vi "FlatSequenceToJSON.vi"(0 "FlatSequence in":refnum<vi>, 1 "Origin Path":path, 5 "Relative Bounds":cluster{"x":i32, "y":i32, "w":i32, "h":i32}, 7 "Current Path":path, 9 "Component Idx":i32, 11 "error in":errorcluster) -> (8 "JSON":string, 15 "error out":errorcluster)   [LabVIEW 2017]
doc: "Converts a flat sequence structure into a JSON"
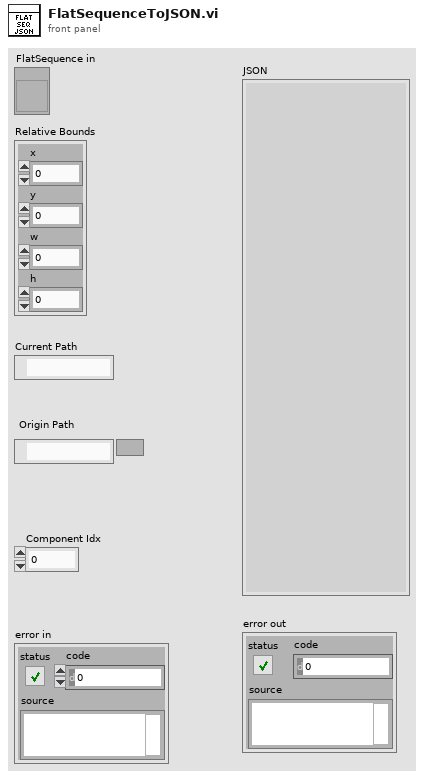
[diagram p1: front panel]
types:
  T1 = typedef "LVRectTypeDef.ctl" = cluster{"Left":i16, "Top":i16, "Right":i16, "Bottom":i16}
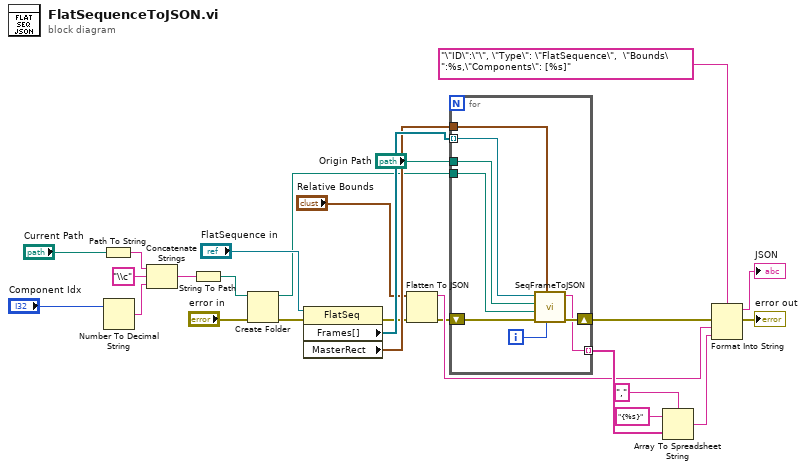
[diagram p0: block diagram]
diagram:
  n1 = Path To String(path="Current Path") -> (string=w15:string)
  n2 = Number To Decimal String(number="Component Idx") -> (decimal integer string=w16:string)  [unwired: 1 in]
  n3 = Concatenate Strings(w15, "\\c" ("string"), w16) -> (w14:string)
  n4 = String To Path(string=w14) -> (path=w13:path)
  n5 = Create Folder(path (use dialog)=w13, error in="error in") -> (created path=w10:path, error out=w11:errorcluster)  [unwired: 1 in, 1 out]
  n6 = property class="FlatSeq"(reference="FlatSequence in", error in=w11) -> (error out=w2:errorcluster, "Frames[]"=w25:refnum<vi>[], "MasterRect"=w20:T1)  [unwired: 1 out]
  n7 = Flatten To JSON(anything="Relative Bounds", error in (no error)=w2) -> (JSON string=w3:string, 11:w1:errorcluster)  [unwired: 1 in]
  n8 = for {
    tunnel: w25 -> [w34] mode=indexing
    shift-right: [w28] -> w23
    shift-left: w1 -> [w30]
    tunnel: w20 -> [w33]
    tunnel: w10 -> [w32]
    tunnel: "Origin Path" -> [w29]
    tunnel: [w27] -> w8 mode=indexing
    i -> [w31]
    n9 = call "SeqFrameToJSON.vi"("Numeric"=w31, "MasterRect"=w33, "error in (no error)"=w30, "created path"=w32, "Origin Path"=w29, "FlatSequenceFrame in"=w34) -> ("error out"=w28:errorcluster, "String"=w27:string)  [unwired: 4 in]
  }
  n10 = Array To Spreadsheet String(delimiter (Tab)=",", array=w8, 3:"{%s}" ("format string")) -> (spreadsheet string=w5:string)
  n11 = Format Into String(format string="\"ID\":\"\", \"Type\": \"FlatSequence\",  \"Bounds\":%s,\"Components\": [%s]", error in=w23, w3, w5) -> (resulting string=→"JSON":string, error out=→"error out":errorcluster)  [unwired: 1 in]
